vi "Auto Step Complete.vi"(0 "L Set Point":dbl, 1 "R Set Point":dbl) -> (6 "Reset":bool, 7 "Distance Reached":bool, 8 "StopStep":bool)   [LabVIEW 2017]
uses:
  Robot Global Data.vi
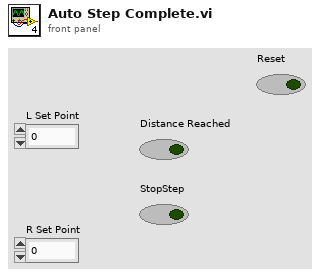
[diagram p1: front panel]
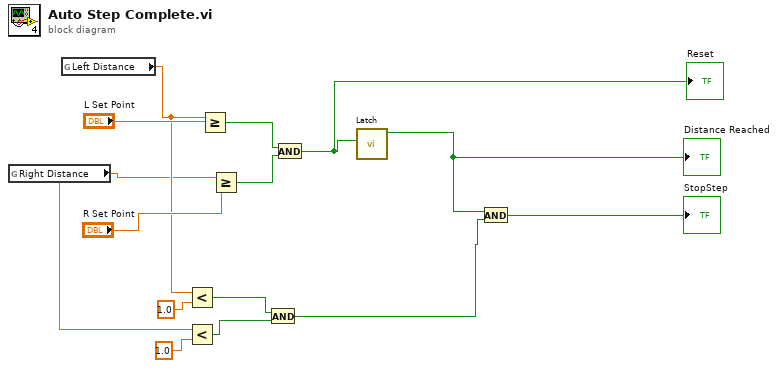
[diagram p0: block diagram]
diagram:
  n1 = global read "Robot Global Data.vi" "Right Distance"() -> (w1:dbl)
  n2 = global read "Robot Global Data.vi" "Left Distance"() -> (w2:dbl)
  n3 = Less?(x=w2, y=1.0) -> (x < y?=w11:bool)
  n4 = Less?(x=w1, y=1.0) -> (x < y?=w12:bool)
  n5 = Greater Or Equal?(x=w2, y="L Set Point") -> (x >= y?=w6:bool)
  n6 = Greater Or Equal?(x=w1, y="R Set Point") -> (x >= y?=w5:bool)
  n7 = And(x=w11, y=w12) -> (x .and. y?=w4:bool)
  n8 = And(x=w6, y=w5) -> (x .and. y?=w3:bool)
  "Reset" <- w3
  n9 = call "Latch.vi"("Input"=w3) -> ("Boolean"=w14:bool)  [unwired: 10 in]
  "Distance Reached" <- w14
  n10 = And(x=w14, y=w4) -> (x .and. y?=→"StopStep":bool)
